vi "Set ETag.vi"(8 "error in (no error)":errorcluster, 10 "ETag":string, 11 "Response in":refnum<class "Response.lvclass">) -> (0 "error out":errorcluster, 3 "Response out":refnum<class "Response.lvclass">)   [LabVIEW 2020, in "HTTP Utils.lvlib" / "Response.lvclass"]
uses:
  Response.lvclass
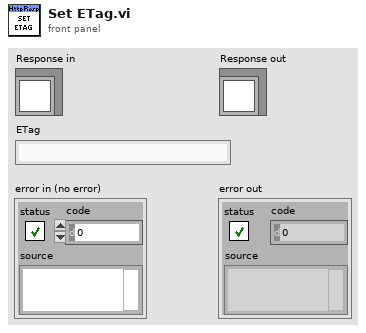
[diagram p1: front panel]
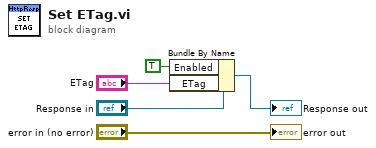
[diagram p0: block diagram]
diagram:
  n1 = Bundle By Name(cluster="Response in", "Enabled"=TRUE ("Cache Params.Enabled"), "ETag"="ETag") -> (→"Response out":refnum<class "Response.lvclass">)
  "error out" <- "error in (no error)"
